vi "Create_Feedforward_File.vi"   [LabVIEW 2013]
uses:
  <vilib>/Utility/file.llb/Write To Spreadsheet File (DBL).vi
  <vilib>/measure/NI_MABase.lvlib
types:
  T1 = cluster{"frequency":dbl, "amplitude":dbl, "phase":dbl}[]
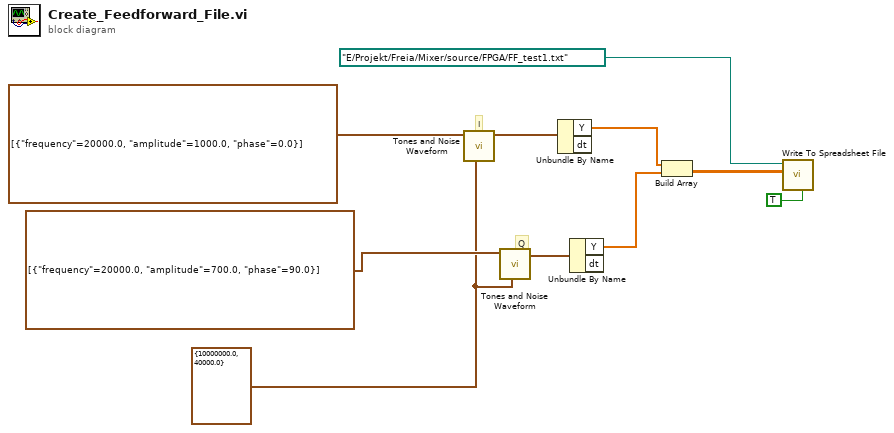
[diagram p0: block diagram]
diagram:
  w8 = cluster{"Fs":dbl, "#s":dbl} {"Fs"=10000000.0, "#s"=40000.0} ("sampling info")
  # "Q"
  # "I"
  n1 = call <vilib>:"Tones and Noise Waveform.vi"("sampling info"=w8, "tones"=T1 [{"frequency"=20000.0, "amplitude"=1000.0, "phase"=0.0}]) -> ("signal out"=w7:waveform(dbl))  [unwired: 8 in, 1 out]
  n2 = call <vilib>:"Tones and Noise Waveform.vi"("sampling info"=w8, "tones"=T1 [{"frequency"=20000.0, "amplitude"=700.0, "phase"=90.0}]) -> ("signal out"=w6:waveform(dbl))  [unwired: 8 in, 1 out]
  n3 = Unbundle By Name(w7) -> ("Y"=w5:dbl[])  [unwired: 1 out]
  n4 = Unbundle By Name(w6) -> ("Y"=w4:dbl[])  [unwired: 1 out]
  n5 = Build Array(w5, w4) -> (w3:dbl[][])
  n6 = call-poly <vilib>:"Write To Spreadsheet File.vi"("transpose? (no:F)"=TRUE, "2D data"=w3, "file path (dialog if empty)"=path "E:/Projekt/Freia/Mixer/source/FPGA/FF_test1.txt") -> ()  [unwired: 5 in, 1 out]
